vi "WriteRowRgbaU32.vi"(8 "error in":errorcluster, 9 "Pixel Row":T1[](array[typedef]), 10 "Row":i32, 11 "Image Reference In":T2) -> (0 "error out":errorcluster, 3 "Image Reference Out":T2)   [LabVIEW 2020, in "OpenLvVision_Image.lvlib" / "DataAccess.lvlib"]
doc: "Write all pixel values in an row."
uses:
  DataAccess.lvlib
  Management/TypeDef/Image.ctl
  TypeDef/RgbaU32.ctl
  <vilib>/Utility/error.llb/Error Cluster From Error Code.vi
  <vilib>/ErrorRing/Error Ring.xnode
  Management/Management.lvlib
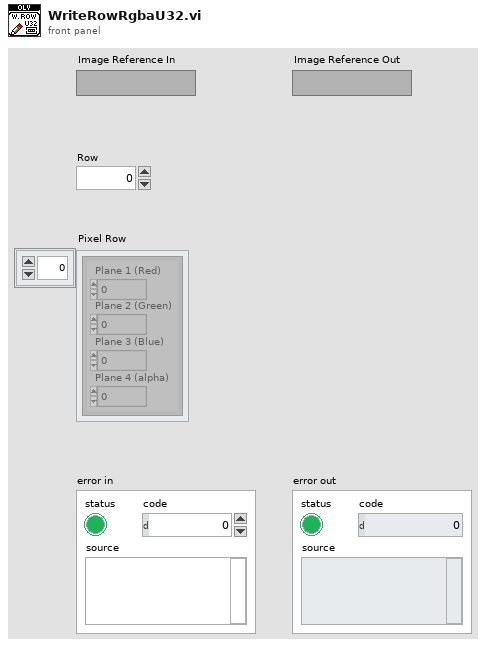
[diagram p1: front panel]
types:
  T1 = typedef "OpenLvVision_Image.lvlib/DataAccess.lvlib/RgbaU32.ctl" = cluster{"Plane 1 (Red)":u8, "Plane 2 (Green)":u8, "Plane 3 (Blue)":u8, "Plane 4 (alpha)":u8}
  T2 = typedef "OpenLvVision_Image.lvlib/Management.lvlib/Image.ctl" = refnum<image>
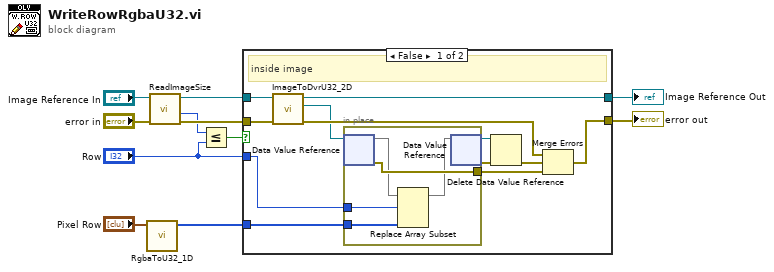
[diagram p0: block diagram]
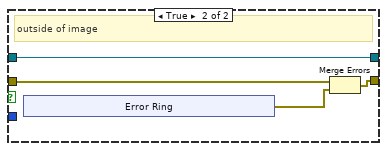
[diagram p2: hidden frame]
diagram:
  n1 = call "RgbaToU32_1D.vi"("Rgba"="Pixel Row") -> ("U32"=w1:u32[])  [unwired: 10 in]
  n2 = call "ReadImageSize.vi"("error in"="error in", "Image Reference In"="Image Reference In") -> ("error out"=w10:errorcluster, "Height"=w3:i32, "Image Reference Out"=w11:T2)  [unwired: 6 in, 1 out]
  n3 = Less Or Equal?(x=w3, y="Row") -> (x <= y?=w5:bool)
  n4 = case shown="False" w5 {
    tunnel: w11 -> [w23 w30]
    tunnel: w10 -> [w22 w32]
    tunnel: [w21 w30] -> w7
    tunnel: [w14 w29] -> w6
    tunnel: "Row" -> [w13 _]
    tunnel: w1 -> [w12 _]
    frame False {
      # "inside image"
      n5 = call "ImageToDvrU32_2D.vi"("error in"=w22, "Image Reference In"=w23) -> ("error out"=w16:errorcluster, "EDVR 2D U32"=w15:refnum<data-value>, "Image Reference Out"=w21:T2)  [unwired: 6 in, 1 out]
      n6 = in-place {
        in-place-border: [w28] -> w19
        in-place-border: w13 -> [w25]
        in-place-border: w12 -> [w24]
        n7 = in-place-dvr #1(w15) -> (w27:u32[][], w28:errorcluster)
        n8 = Replace Array Subset(array=w27, new element=w24, index (row)=w25) -> (w26:u32[][])  [unwired: 1 in]
        n9 = in-place-dvr #1(w26) -> (w17:refnum<data-value>, w18:errorcluster)
      }
      n10 = Delete Data Value Reference(data value reference=w17, error in=w18) -> (error out=w20:errorcluster)  [unwired: 1 out]
      n11 = Merge Errors(w16, w20, w19) -> (w14:errorcluster)
    }
    frame True {
      # "outside of image"
      n12 = xnode "Error Ring"() -> ("error out"=w31:errorcluster)
      n13 = Merge Errors(w32, w31) -> (w29:errorcluster)
    }
  }
  "error out" <- w6
  "Image Reference Out" <- w7
